vi "Set Parameter Value by Name (Stringl).vi"(0 "Parameter Array":string[](array[string]), 5 "Parameter Name":string, 9 "String":string, 12 "Create if not found (T)":bool=TRUE, 13 "Override if found (T)":bool=TRUE) -> (4 "Parameter Array Out":string[](array[string]), 8 "Found?":bool, 10 "Value is there":bool, 15 "Created New":bool)   [LabVIEW 2014]
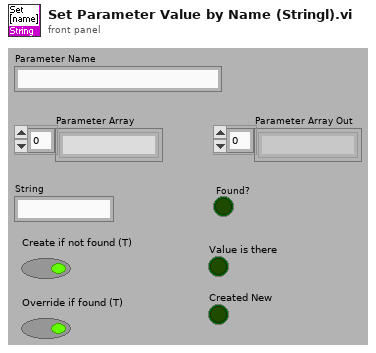
[diagram p1: front panel]
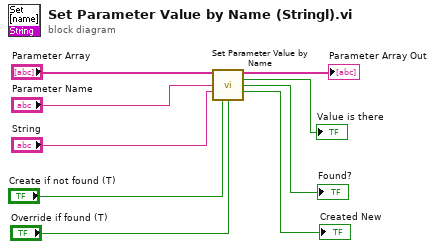
[diagram p0: block diagram]
diagram:
  n1 = call "Set Parameter Value by Name.vi"("Parameter Array"="Parameter Array", "Parameter Name"="Parameter Name", "flattened value"="String", "Create if not found"="Create if not found (T)", "Override if found"="Override if found (T)") -> ("Parameter Array Out"=→"Parameter Array Out":string[], "Value is there"=→"Value is there":bool, "Found?"=→"Found?":bool, "Created New"=→"Created New":bool)  [unwired: 7 in]
